vi "FileMultipleBackup.vi"(9 "Backup Extention (.bak)":string=".bak", 10 "Number of Backups":i32=10, 11 "File path":path) -> (3 "File path out":path)   [LabVIEW 2020]
uses:
  <vilib>/regexp/Match Regular Expression.xnode
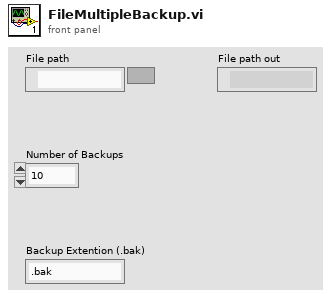
[diagram p1: front panel]
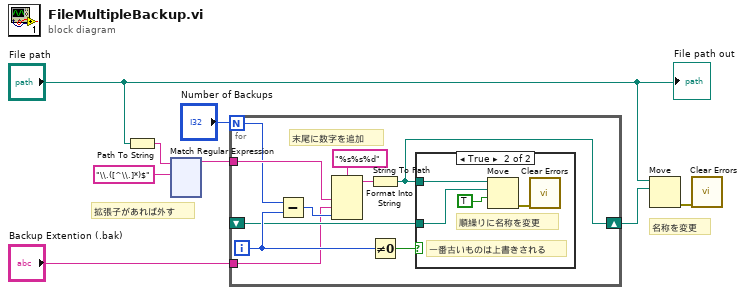
[diagram p0: block diagram]
diagram:
  # "拡張子があれば外す"
  # "名称を変更"
  n1 = Path To String(path="File path") -> (string=w6:string)
  n2 = xnode "Match Regular Expression"("input string"=w6, "regular expression"="\\.([^\\.]*)$") -> ("before match"=w4:string)  [unwired: 4 in, 4 out]
  n3 = for {
    N: "Number of Backups" -> [w15]
    tunnel: w4 -> [w18]
    shift-right: [w12] -> w3
    shift-left: _ -> [w11]
    tunnel: "Backup Extention (.bak)" -> [w9]
    i -> [w14]
    # "末尾に数字を追加"
    n4 = Subtract(x=w15, y=w14) -> (x-y=w10:i32)
    n5 = Format Into String(format string="%s%s%d", w18, w9, w10) -> (resulting string=w16:string)  [unwired: 2 in, 1 out]
    n6 = String To Path(string=w16) -> (path=w12:path)
    n7 = Not Equal To 0?(x=w14) -> (x != 0?=w13:bool)
    n8 = case shown="True" w13 {
      tunnel: w12 -> [_ w21]
      tunnel: w11 -> [_ w22]
      frame False {
      }
      frame True {
        # "一番古いものは上書きされる"
        # "順繰りに名称を変更"
        n9 = Move(source path=w21, 9:TRUE ("overwrite (F)"), 10:w22) -> (error out=w19:errorcluster)  [unwired: 2 in, 2 out]
        n10 = call <vilib>:"Clear Errors.vi"("error in (no error)"=w19) -> ()  [unwired: 5 in, 2 out]
      }
    }
  }
  n11 = Move(source path="File path", 10:w3) -> (error out=w7:errorcluster)  [unwired: 3 in, 2 out]
  n12 = call <vilib>:"Clear Errors.vi"("error in (no error)"=w7) -> ()  [unwired: 5 in, 2 out]
  "File path out" <- "File path"
